vi "Tree.vi"   [LabVIEW 2018]
uses:
  <vilib>/National Instruments/Tree Map/Tree Map.lvlib
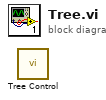
[diagram p0: block diagram]
diagram:
  n1 = call <vilib>:"Tree Control.vi"() -> ()  [unwired: 12 in]
